vi "Set Voltage.vi"(8 "error in":errorcluster, 10 "Voltage":dbl, 11 "Power Supply in":refnum<class "Power Supply.lvclass">) -> (0 "error out":errorcluster, 3 "Power Supply out":refnum<class "Power Supply.lvclass">)   [LabVIEW 2018, in "Power Supply.lvlib" / "Power Supply.lvclass"]
doc: "This VI stores the Voltage settings and then sends all settings to the power supply."
uses:
  Power Supply.lvclass
  Power Supply.lvclass/Power Supply.ctl
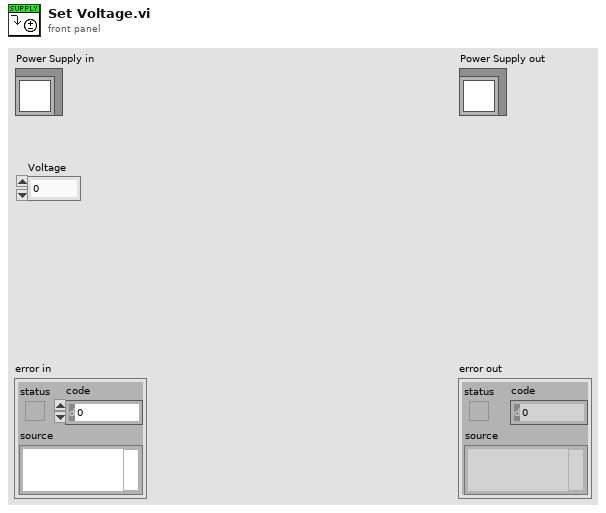
[diagram p1: front panel]
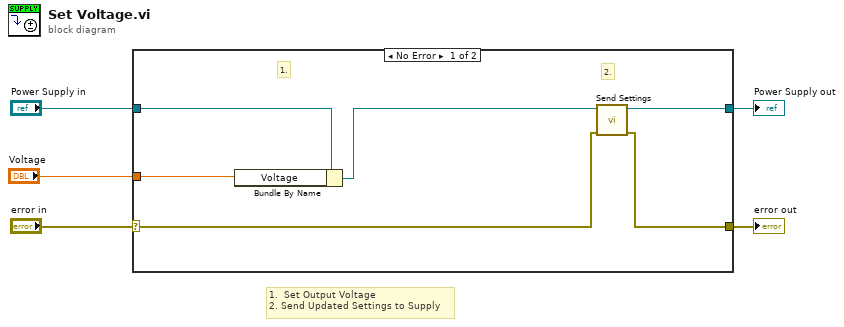
[diagram p0: block diagram]
diagram:
  # "1.  Set Output Voltage\n2. Send Updated Settings to Supply"
  n1 = case shown="No Error" "error in" {
    selector: "error in" -> [w7 w13]
    tunnel: [w6 w13] -> w4
    tunnel: [w10 w12] -> w2
    tunnel: "Power Supply in" -> [w11 w12]
    tunnel: "Voltage" -> [w8 _]
    frame No Error {
      # "2."
      # "1."
      n2 = Bundle By Name(cluster=w11, "Voltage"=w8) -> (w9:refnum<class "Power Supply.lvclass">)
      n3 = call-dynamic "Send Settings.vi"("error in (no error)"=w7, "Power Supply in"=w9) -> ("error out"=w6:errorcluster, "Power Supply out"=w10:refnum<class "Power Supply.lvclass">)  [unwired: 8 in]
    }
    frame Error {
    }
  }
  "error out" <- w4
  "Power Supply out" <- w2
